vi "Ajutator.vi"(1 "kxk":dbl, 2 "Input":dbl[][](array[numeric]) format="%#_10f") -> (0 "Output":dbl[][](array[numeric]) format="%#_10f")   [LabVIEW 2018]
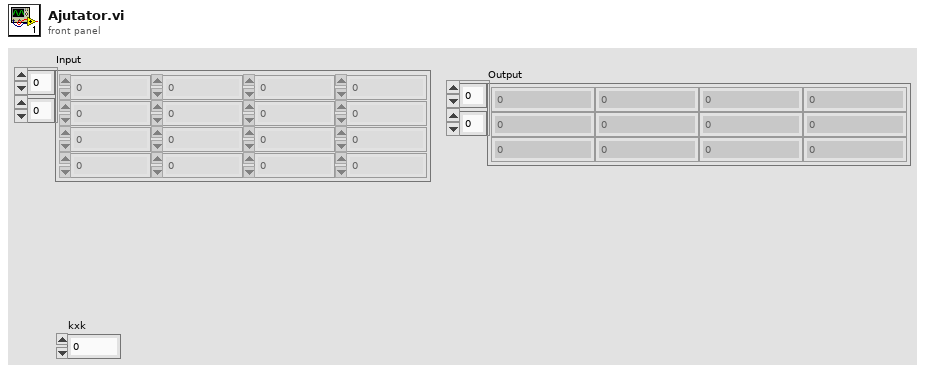
[diagram p1: front panel]
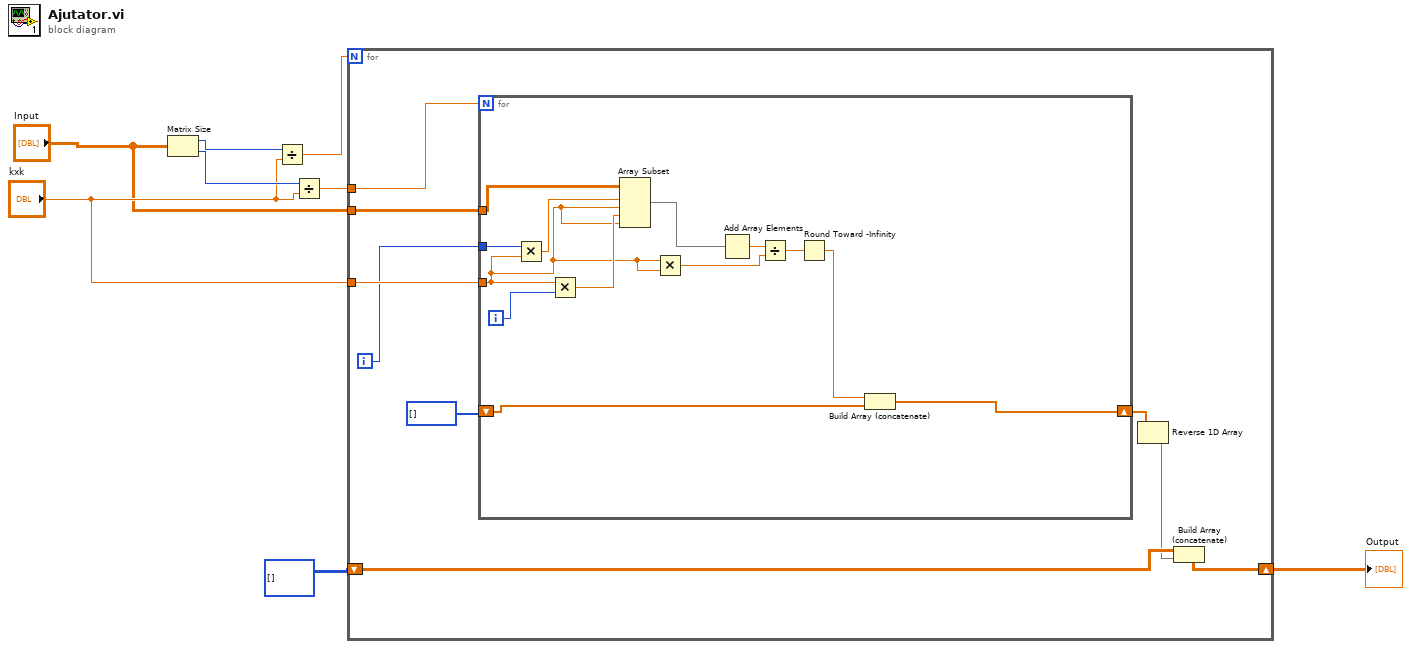
[diagram p0: block diagram]
diagram:
  n1 = Matrix Size(0:"Input") -> (1:w8:i32, 2:w6:i32)
  n2 = Divide(x=w8, y="kxk") -> (x/y=w7:dbl)
  n3 = Divide(x=w6, y="kxk") -> (x/y=w5:dbl)
  n4 = for {
    N: w7 -> [_]
    tunnel: w5 -> [w17]
    tunnel: "Input" -> [w16]
    tunnel: "kxk" -> [w15]
    shift-right: [w12] -> w2
    shift-left: i32[][] [] -> [w11]
    i -> [w14]
    n5 = for {
      N: w17 -> [_]
      tunnel: w16 -> [w30]
      tunnel: w15 -> [w23]
      tunnel: w14 -> [w28]
      shift-right: [w18] -> w10
      shift-left: i32[] [] -> [w20]
      i -> [w29]
      n6 = Multiply(x=w28, y=w23) -> (x*y=w27:dbl)
      n7 = Multiply(x=w23, y=w29) -> (x*y=w26:dbl)
      n8 = Array Subset(array=w30, index (row)=w27, length (row)=w23, index (col)=w26, length (col)=w23) -> (w25:dbl[][])
      n9 = Multiply(x=w23, y=w23) -> (x*y=w22:dbl)
      n10 = Add Array Elements(numeric array=w25) -> (sum=w24:dbl)
      n11 = Divide(x=w24, y=w22) -> (x/y=w21:dbl)
      n12 = Round Toward -Infinity(1:w21) -> (0:w19:dbl)
      n13 = Build Array (concatenate)(w19, w20) -> (w18:dbl[])
    }
    n14 = Reverse 1D Array(array=w10) -> (reversed array=w9:dbl[])
    n15 = Build Array (concatenate)(w11, w9) -> (w12:dbl[][])
  }
  "Output" <- w2
